vi "Write Shutdown Timeout (ms).vi"(8 "error in (no error)":errorcluster, 10 "Shutdown Timeout (ms)":i32=5000, 11 "AdvancedActor in":refnum<class "AdvancedActor.lvclass">) -> (0 "error out":errorcluster, 3 "AdvancedActor out":refnum<class "AdvancedActor.lvclass">)   [LabVIEW 2020, in "MGI-Panel Actor.lvlib" / "AdvancedActor.lvlib" / "AdvancedActor.lvclass"]
uses:
  AdvancedActor.lvclass
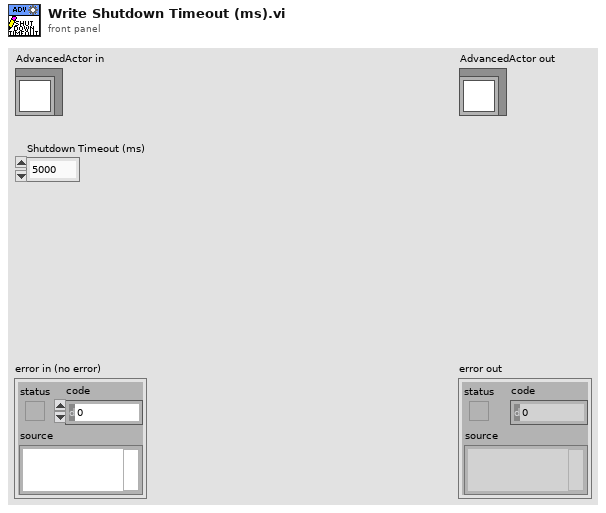
[diagram p1: front panel]
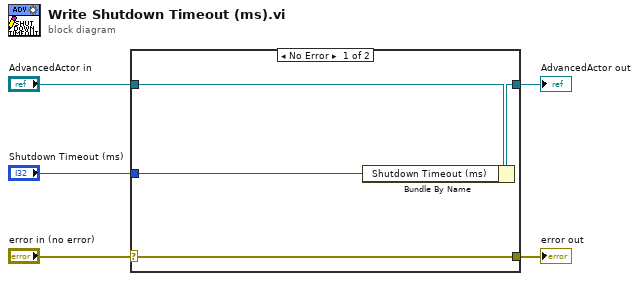
[diagram p0: block diagram]
diagram:
  n1 = case shown="No Error" "error in (no error)" {
    selector: "error in (no error)" -> [w9 w10]
    tunnel: [w9 w10] -> w4
    tunnel: [w7 w11] -> w2
    tunnel: "AdvancedActor in" -> [w8 w11]
    tunnel: "Shutdown Timeout (ms)" -> [w6 _]
    frame No Error {
      n2 = Bundle By Name(cluster=w8, "Shutdown Timeout (ms)"=w6) -> (w7:refnum<class "AdvancedActor.lvclass">)
    }
    frame Error {
    }
  }
  "error out" <- w4
  "AdvancedActor out" <- w2
